vi "VerifyDeviceIsPresent.vi"(8 "Error In":errorcluster, 11 "Serial Number in":string) -> (0 "Error Out":errorcluster, 3 "Present?":bool)   [LabVIEW 2018, in "ThorlabsLabJack.lvlib" / "ThorlabsLabJack.lvclass"]
uses:
  ThorlabsLabJack.lvclass
  C:/Projects/LabVIEW/In-Progress/Chetan Malpure/Axis/Thorlabs LabJack/Drivers/Thorlabs.MotionControl.DeviceManagerCLI.dll
  Drivers/Thorlabs.MotionControl.DeviceManagerCLI.dll
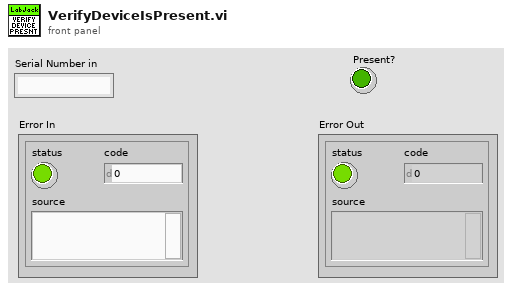
[diagram p1: front panel]
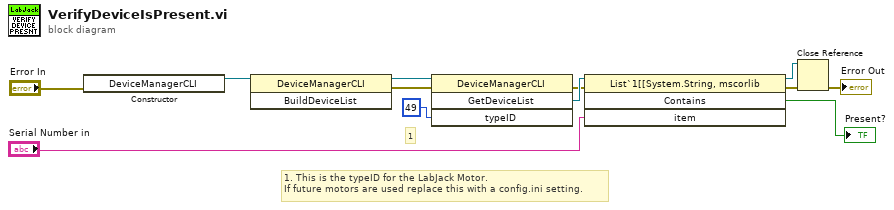
[diagram p0: block diagram]
diagram:
  # "1. This is the typeID for the LabJack Motor.\nIf future motors are used replace this with a config.ini setting."
  # "1"
  n1 = constructor class="DeviceManagerCLI"(error in="Error In") -> (reference out=w3:refnum<k24>)  [unwired: 2 in, 2 out]
  n2 = invoke class="DeviceManagerCLI" method="BuildDeviceList"(reference=w3) -> (reference out=w5:refnum<k24>, error out=w11:errorcluster)  [unwired: 2 in, 1 out]
  n3 = invoke class="DeviceManagerCLI" method="GetDeviceList"(reference=w5, error in=w11, "typeID"=49) -> (error out=w8:errorcluster, "GetDeviceList"=w9:refnum<k24>)  [unwired: 1 in, 2 out]
  n4 = invoke class="List`1[[System.String, mscorlib" method="Contains"(reference=w9, error in=w8, "item"="Serial Number in") -> (reference out=w6:refnum<k24>, error out=w7:errorcluster, "Contains"=→"Present?":bool)  [unwired: 1 in, 1 out]
  n5 = Close Reference(reference=w6, error in (no error)=w7) -> (error out=→"Error Out":errorcluster)
